vi "Update Power Display.vi"(9 "Power":dbl, 10 "Channel":u8, 11 "Array Refnum":refnum<vi>) -> ()   [LabVIEW 2019, in "UI.lvlib"]
uses:
  UI.lvlib
  Channel Controls.ctl
  Channel Control.ctl
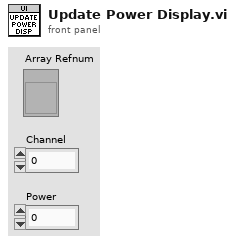
[diagram p1: front panel]
types:
  T1 = typedef "UI.lvlib/Channel Controls.ctl" = T2[]
  T2 = typedef "UI.lvlib/Channel Control.ctl" = cluster{"Power":dbl, "Frequency":dbl, "PLL":bool, "A/B":bool}
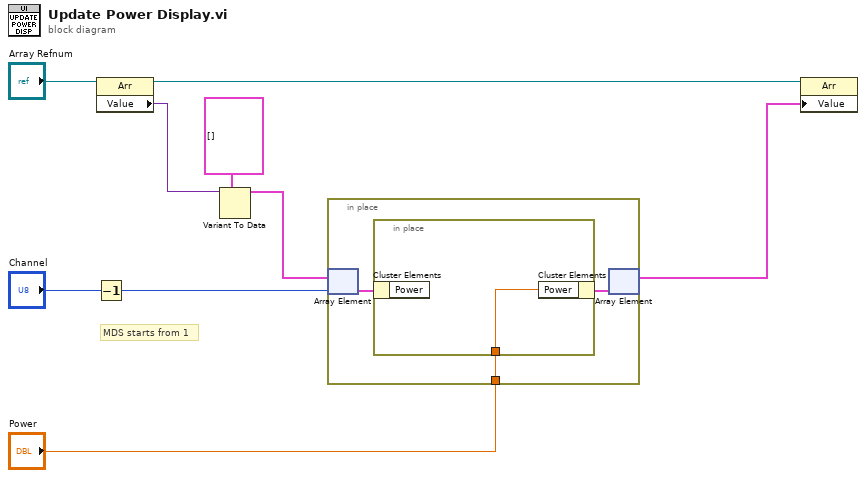
[diagram p0: block diagram]
diagram:
  # "MDS starts from 1"
  n1 = Decrement(x="Channel") -> (x-1=w1:u8)
  n2 = property class="Arr"(reference="Array Refnum") -> (reference out=w7:refnum<vi>, "Value"=w4:variant)  [unwired: 1 in, 1 out]
  n3 = Variant To Data(type=T1 [] ("Channels"), Variant=w4) -> (data=w3:T1)  [unwired: 1 in, 1 out]
  n4 = in-place {
    in-place-border: "Power" -> [w12]
    n5 = in-place-array #1(w3, w1) -> (w11:T2)
    n6 = in-place {
      in-place-border: w12 -> [w13]
      n7 = in-place-cluster #2(w11) -> ()  [unwired: 1 out]
      n8 = in-place-cluster #2("Power"=w13) -> (w10:T2)
    }
    n9 = in-place-array #1(w10) -> (w9:T1)  [unwired: 1 out]
  }
  n10 = property class="Arr"(reference=w7, "Value"=w9) -> ()  [unwired: 1 in, 2 out]
